vi "RichToFlatcif_plugincore_StartRequest.vi"(5 "OutputClusterType":T1, 11 "InputCluster":T2) -> (3 "OutputCluster":T1)   [LabVIEW 2021, in "CIFCorePlugin_server.lvlib"]
uses:
  CIFCorePlugin_server.lvlib
  cif_plugincore_StartRequest.ctl
  cif_plugincore_StartRequest_Flat.ctl
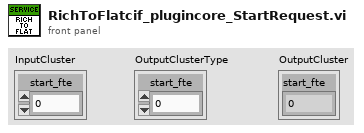
[diagram p1: front panel]
types:
  T1 = typedef "CIFCorePlugin_server.lvlib/cif_plugincore_StartRequest_Flat.ctl" = cluster{"start_fte":i64}
  T2 = typedef "CIFCorePlugin_server.lvlib/cif_plugincore_StartRequest.ctl" = cluster{"start_fte":i64}
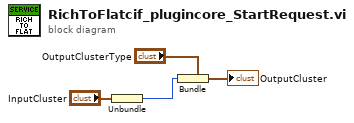
[diagram p0: block diagram]
diagram:
  n1 = Unbundle "Unbundle"("InputCluster") -> ("start_fte"=w1:i64)
  n2 = Bundle "Bundle"(cluster="OutputClusterType", "start_fte"=w1) -> (→"OutputCluster":T1)
